vi "GE 5565PIORC.VISA.Move In.String (U8).vi"(7 "address space":T1=1 items=["VXI/VME A16"=1, "VXI/VME A24"=2, "VXI/VME A32"=3, "VXI/VME A64"=4, "PXI Memory Allocations"=9, "PXI Configuration"=10, "PXI BAR0"=11, "PXI BAR1"=12, "PXI BAR2"=13, "PXI BAR3"=14, "PXI BAR4"=15, "PXI BAR5"=16], 8 "error in (no error)":errorcluster, 9 "count":u32, 10 "offset":u32, 11 "GE 5565PIORC in":refnum<class "GE 5565PIORC.lvclass">) -> (0 "error out":errorcluster, 1 "data out":string, 3 "GE 5565PIORC out":refnum<class "GE 5565PIORC.lvclass">)   [LabVIEW 2016, in "GE 5565PIORC.lvclass"]
uses:
  GE 5565PIORC.lvclass
  <vilib>/Instr/_visa.llb/VISA Register Access Address Space.ctl
  GE 5565PIORC.lvclass/GE 5565PIORC.ctl
  <vilib>/Utility/error.llb/Error Cluster From Error Code.vi
  visa32.dll
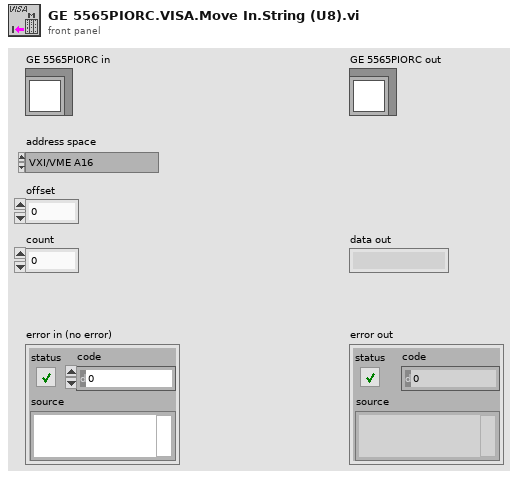
[diagram p1: front panel]
types:
  T1 = typedef "VISA Register Access Address Space.ctl" = u16
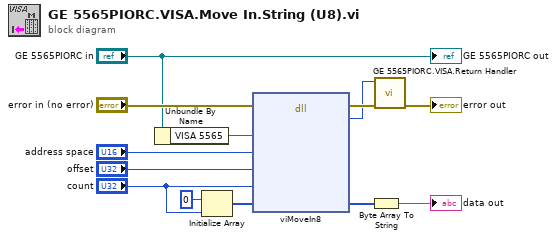
[diagram p0: block diagram]
diagram:
  n1 = Unbundle By Name("GE 5565PIORC in") -> ("VISA 5565"=w2:refnum<visa-resource-name>)
  n2 = Initialize Array(u8 0 ("element"), "count") -> (w9:u8[])
  n3 = dll-call lib="visa32.*" fn="viMoveIn8"(error in="error in (no error)", "session"=w2, "address space"="address space", "offset"="offset", "size"="count", "data"=w9) -> (error out=w8:errorcluster, "return type"=w6:i32, "data"=w4:u8[])  [unwired: 6 in, 1 out]
  n4 = Byte Array To String(unsigned byte array=w4) -> (string=→"data out":string)
  n5 = call "GE 5565PIORC.VISA.Return Handler.vi"("error in (no error)"=w8, "VISA return value"=w6) -> ("error out"=→"error out":errorcluster)  [unwired: 9 in]
  "GE 5565PIORC out" <- "GE 5565PIORC in"
